vi "GL302 Status.vi"(10 "bytes to read":u32) -> (1 "Numeric":u32, 2 "String":string)   [LabVIEW 2014]
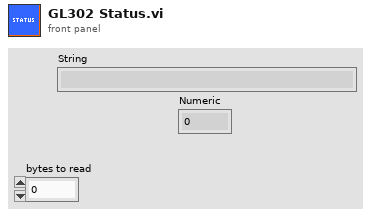
[diagram p1: front panel]
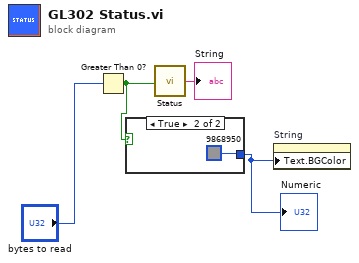
[diagram p0: block diagram]
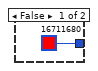
[diagram p2: hidden frame]
diagram:
  n1 = Greater Than 0?(x="bytes to read") -> (x > 0?=w4:bool)
  n2 = case shown="True" w4 {
    tunnel: [u32 16711680 u32 9868950] -> w1
    frame False {
    }
    frame True {
    }
  }
  "Numeric" <- w1
  n3 = call "Status.vi"("Status"=w4) -> ("String"=→"String":string)
  n4 = property on="String" class="Str"("Text.BGColor"=w1) -> ()  [unwired: 2 in, 2 out]
